vi "SetDacValueMan_individualDAC_vnico.vi"(1 "DAC":bool, 2 "DAC write (mV)":dbl, 3 "DAC number":u8=2 min=1 max=8, 4 "RS232/ Optical Fiber":refnum<visa-resource-name>="COM2") -> (0 "DAC read (mV)":dbl)   [LabVIEW 2011]
panel:
  # "Dilution room :  COM2"
  # "Set dac value manually\nDac value is swept safely"
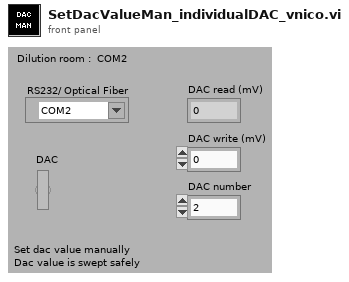
[diagram p1: front panel]
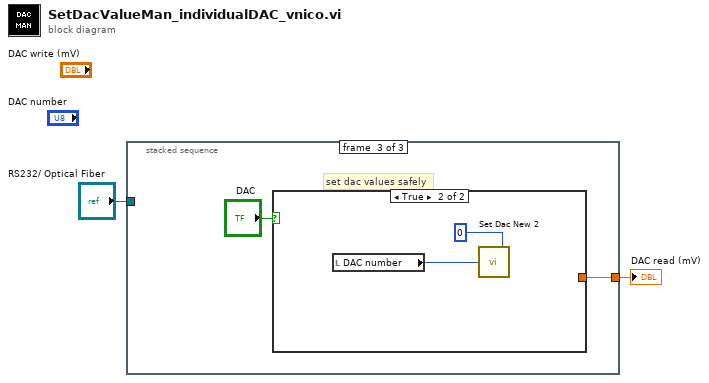
[diagram p0: block diagram]
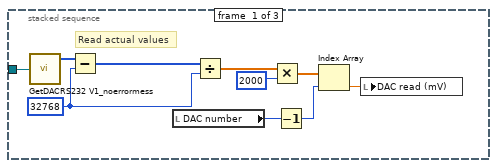
[diagram p2: hidden frame]
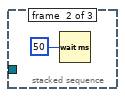
[diagram p3: hidden frame]
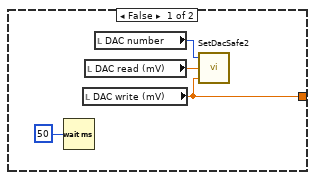
[diagram p4: hidden frame]
diagram:
  n1 = stacked-sequence {
    tunnel: "RS232/ Optical Fiber" -> [w4 _ _]
    tunnel: [_ _ w14] -> w1
    frame #0 {
      w10 = 32768
      # "Read actual values"
      n2 = call "GetDACRS232 V1_noerrormess.vi"("VISA resource name IN"=w4) -> ("DAC data out\n(hexadecimaal)"=w3:u16[])  [unwired: 2 in, 2 out]
      n3 = Subtract(x=w3, y=w10) -> (x-y=w9:i32[])
      n4 = local read "DAC number"() -> (w6:u8)
      n5 = Divide(x=w9, y=w10) -> (x/y=w11:dbl[])
      n6 = Multiply(x=w11, y=2000) -> (x*y=w8:dbl[])
      n7 = Decrement(x=w6) -> (x-1=w5:u8)
      n8 = Index Array(array=w8, index=w5) -> (element=w7:dbl)
      n9 = local write "DAC read (mV)"(w7) -> ()
    }
    frame #1 {
      n10 = Wait (ms)(milliseconds to wait=50) -> ()  [unwired: 1 out]
    }
    frame #2 {
      # "set dac values safely"
      n11 = case shown="True" "DAC" {
        tunnel: [w16 _] -> w14
        frame False {
          n12 = Wait (ms)(milliseconds to wait=50) -> ()  [unwired: 1 out]
          n13 = local read "DAC write (mV)"() -> (w16:dbl)
          n14 = local read "DAC read (mV)"() -> (w17:dbl)
          n15 = local read "DAC number"() -> (w18:u8)
          n16 = call "SetDacSafe2.vi"("New Value (mV)"=w16, "Actual Value DAC (mV)"=w17, "DAC Nr."=w18) -> ()  [unwired: 1 out]
        }
        frame True {
          n17 = local read "DAC number"() -> (w20:u8)
          n18 = call "Set Dac New 2.vi"("DATA (V)"=0, "DAC nr"=w20) -> ()
        }
      }
    }
  }
  "DAC read (mV)" <- w1
